vi "Capture Template Image.vi"(5 "Main_Gray":T1, 6 "RGB?Color":bool, 7 "Main_RGB":T1, 8 "error in":errorcluster, 10 "Color Plane":i32(ring)=5 items=["Red", "Green", "Blue", "Hue", "Saturation", "Luminance", "Value", "Intensity"], 11 "Template Path":path) -> (0 "error out":errorcluster, 1 "Main_Gray Out":T1)   [LabVIEW 2020]
uses:
  <vilib>/vision/Image Controls.llb/IMAQ Image.ctl
  <vilib>/vision/NI_Vision_Development_Module.lvlib
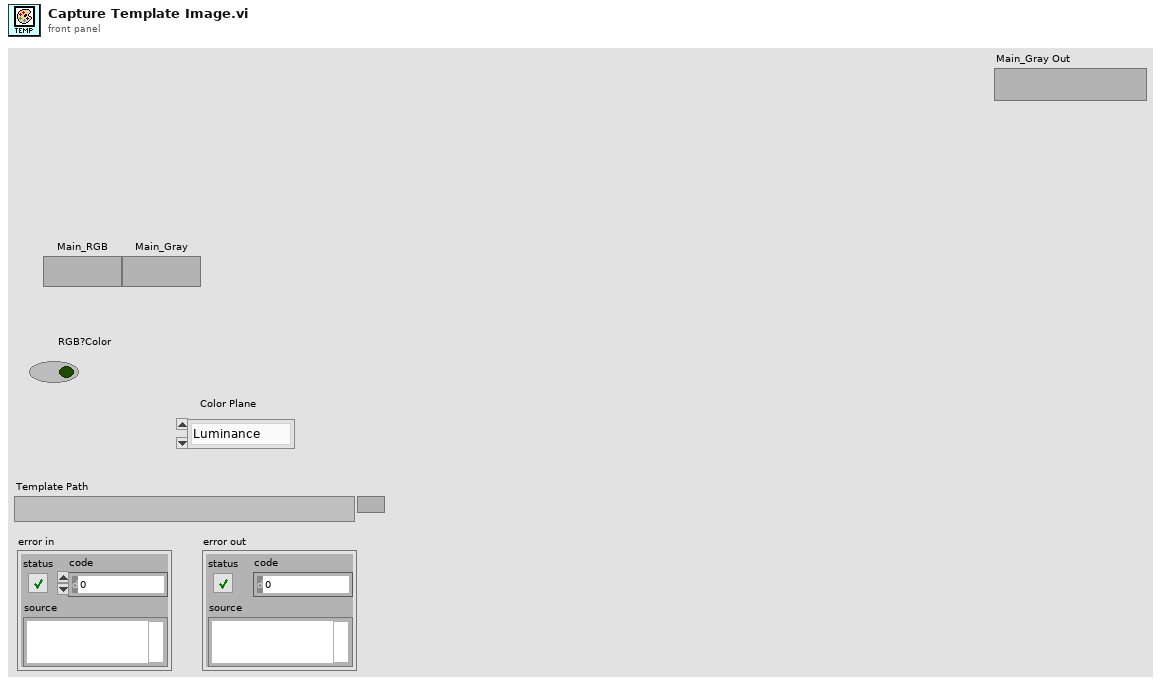
[diagram p1: front panel]
types:
  T1 = typedef "IMAQ Image.ctl" = refnum<image>
  T2 = typedef "Image Type" = u32
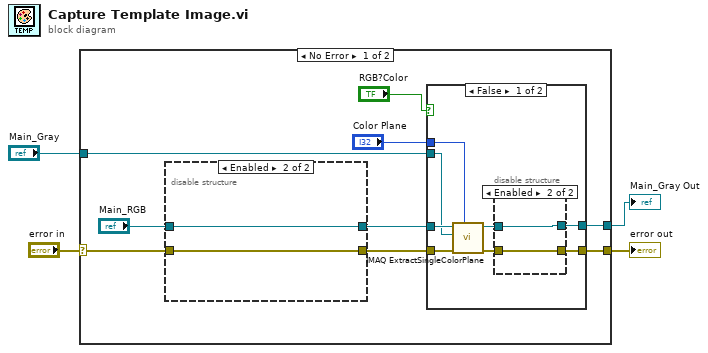
[diagram p0: block diagram]
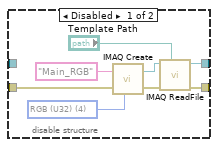
[diagram p2: hidden frame]
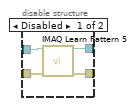
[diagram p3: hidden frame]
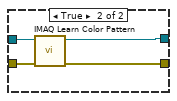
[diagram p4: hidden frame]
diagram:
  n1 = case shown="No Error" "error in" {
    selector: "error in" -> [w7 w42]
    tunnel: [w10 w42] -> w1
    tunnel: [w9 _] -> w2
    tunnel: "Main_Gray" -> [w5 _]
    frame No Error {
      n2 = disable-structure shown="Enabled" {
        disable-tunnel: [w21 w23] -> w13
        disable-tunnel: [w20 w22] -> w11
        disable-tunnel: w7 -> [w19 w23]
        disable-tunnel: "Main_RGB" -> [_ w22]
        frame Disabled {
          w16 = T2 4 items=["Grayscale (U8)", "Grayscale (I16)", "Grayscale (SGL)", "Complex (CSG)", "RGB (U32)", "HSL (U32)", "RGB (U64)", "Grayscale (U16)"] ("Image Type")
          n3 = call "IMAQ Create"("Image Name"="Main_RGB", "Image Type"=w16, "error in (no error)"=w19) -> ("New Image"=w14:T1, "error out"=w17:errorcluster)  [unwired: 2 in]
          n4 = call "IMAQ ReadFile"("File Path"="Template Path", "error in (no error)"=w17, "Image"=w14) -> ("error out"=w21:errorcluster, "Image Out"=w20:T1)  [unwired: 4 in, 3 out]
        }
        frame Enabled {
        }
      }
      n5 = case shown="False" "RGB?Color" {
        tunnel: w13 -> [w30 w38]
        tunnel: "Color Plane" -> [w29 _]
        tunnel: w11 -> [w28 w39]
        tunnel: [w26 w40] -> w10
        tunnel: [w25 w41] -> w9
        tunnel: w5 -> [w24 _]
        frame False {
          n6 = call "IMAQ ExtractSingleColorPlane"("Color Plane"=w29, "error in (no error)"=w30, "Image Dst"=w24, "Image Src"=w28) -> ("error out"=w27:errorcluster, "Image Dst Out"=w31:T1)  [unwired: 6 in]
          n7 = disable-structure shown="Enabled" {
            disable-tunnel: w31 -> [w35 w37]
            disable-tunnel: w27 -> [w34 w36]
            disable-tunnel: [w33 w36] -> w26
            disable-tunnel: [w32 w37] -> w25
            frame Disabled {
              n8 = call "IMAQ Learn Pattern 5"("Image"=w35, "error in (no error)"=w34) -> ("Template Image Out"=w32:T1, "error out"=w33:errorcluster)  [unwired: 11 in, 1 out]
            }
            frame Enabled {
            }
          }
        }
        frame True {
          n9 = call "IMAQ Learn Color Pattern"("error in (no error)"=w38, "Image"=w39) -> ("error out"=w40:errorcluster, "Template Image Out"=w41:T1)  [unwired: 8 in]
        }
      }
    }
    frame Error {
    }
  }
  "error out" <- w1
  "Main_Gray Out" <- w2
